vi "CRYPer.Rub& Buzz.vi"(4 "response":dbl[](array[numeric]), 5 "stimulus":dbl[](array[numeric]), 8 "cycle":dbl, 9 "frequency":dbl) -> (3 "out Y":dbl)   [LabVIEW 2013]
panel:
  in  "response 2":dbl[](array[numeric])
  in  "stimulus 2":dbl[](array[numeric])
  out "Array":dbl[](array[numeric])
  out "Version":i32
  out "Real matrix":dbl[][](array[numeric])
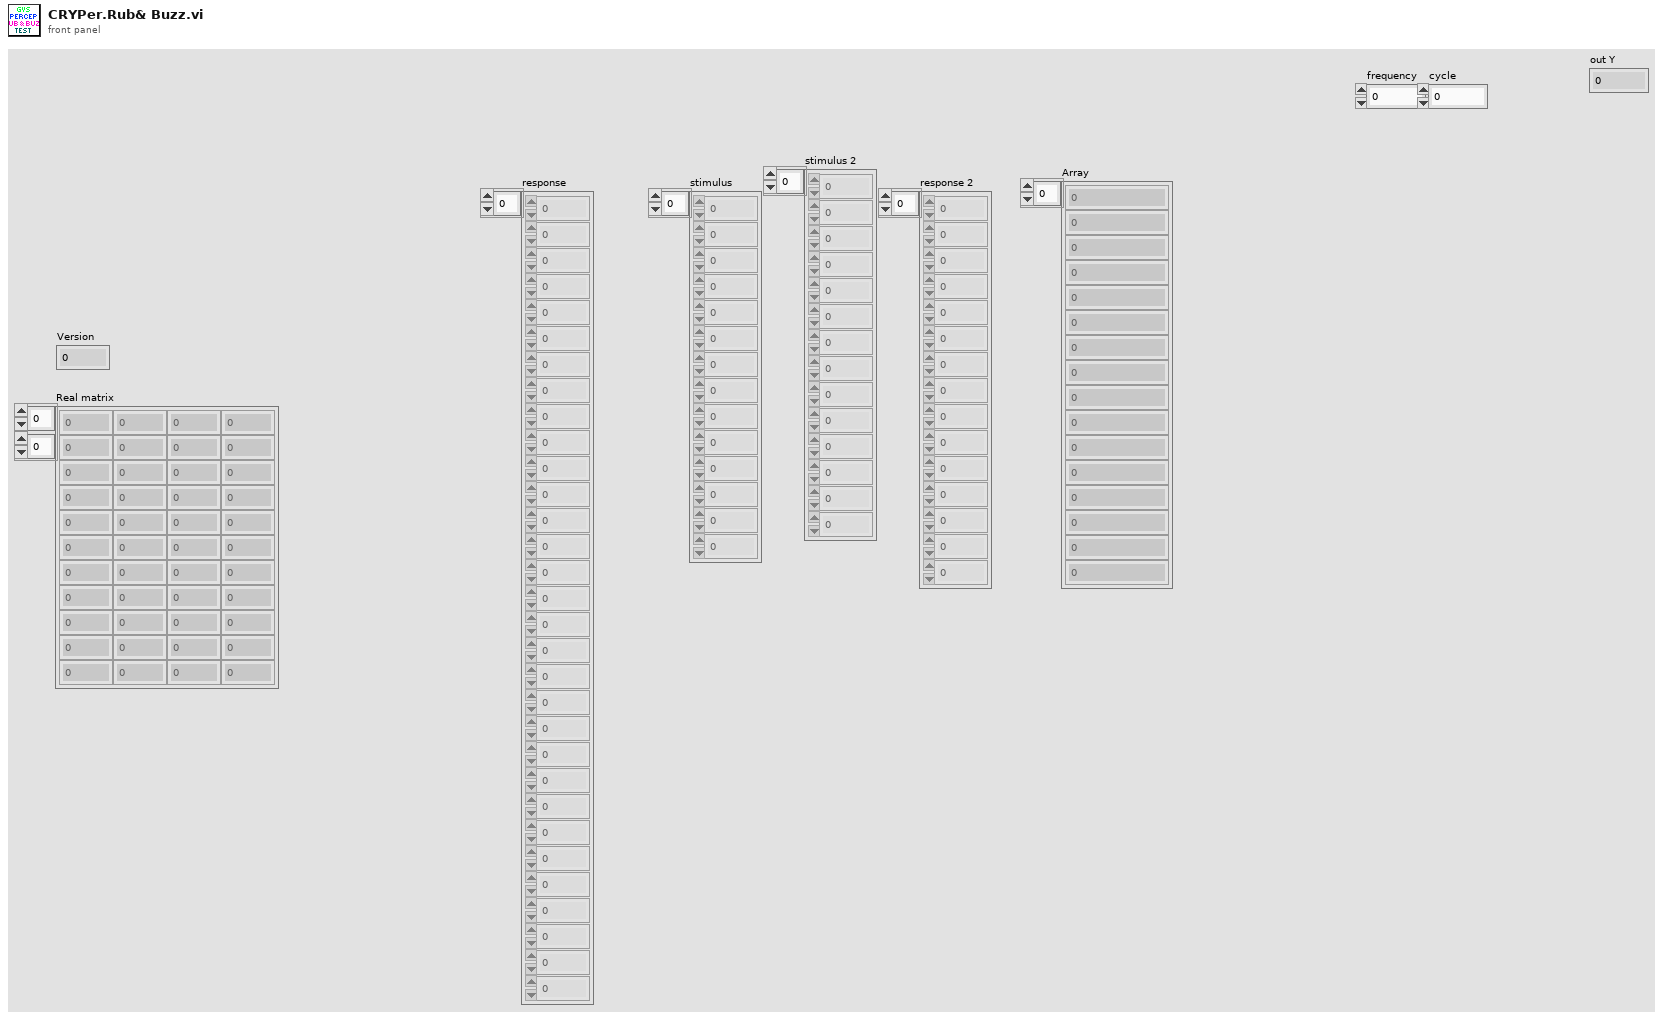
[diagram p1: front panel]
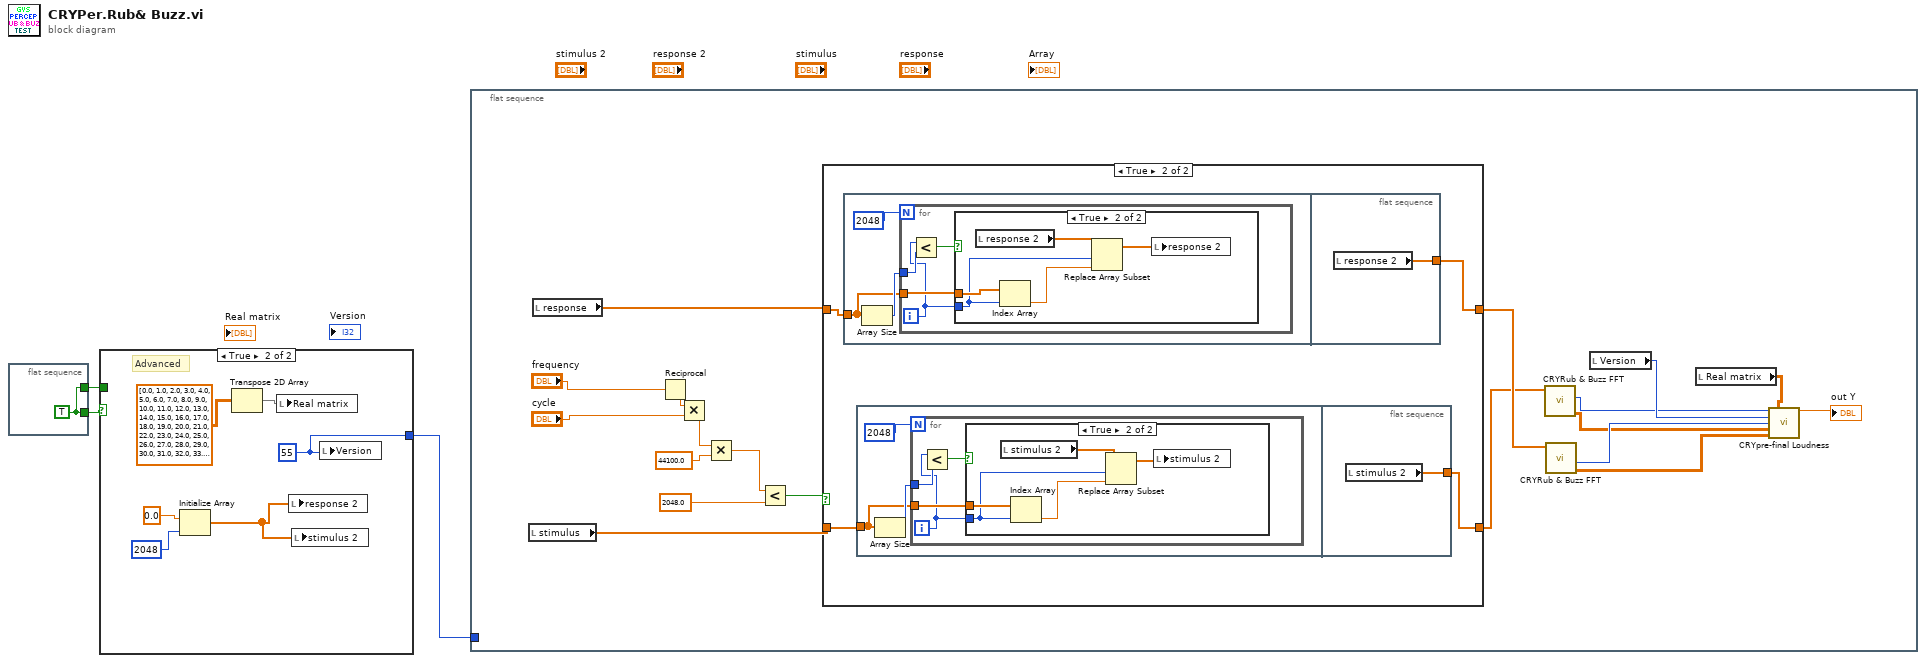
[diagram p0: block diagram]
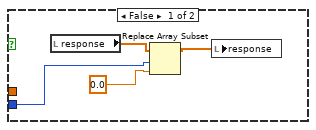
[diagram p3: hidden frame]
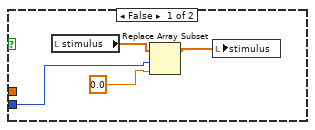
[diagram p4: hidden frame]
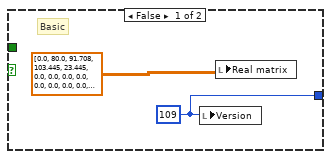
[diagram p5: hidden frame]
diagram:
  n1 = flat-sequence {
    tunnel: [w4] -> w3
    tunnel: [w4] -> w2
    frame #0 {
      w4 = TRUE
    }
  }
  n2 = case shown="True" w3 {
    tunnel: [w6 w12] -> w1
    tunnel: w2 -> [_ _]
    frame False {
      w6 = 109
      # "Basic"
      n3 = local write "Version"(w6) -> ()
      n4 = local write "Real matrix"(dbl[][] [[0.0, 80.0, 91.708, 103.445, 23.445, 0.0, 0.0, 0.0, 0.0, 0.0, 0.0, 0.0, 0.0, 0.0], [1.0, 103.445, 115.216, 127.023, 23.577, 0.0, 0.0, 0.0, 0.0, 0.0, 0.0, 0.0, 0.0, 0.0], [2.0, 127.023, 138.87, 150.762, 23.739, 0.0, 0.0, 0.0, 0.0, 0.0, 0.0, 0.0, 0.0, 0.0], [3.0, 150.762, 162.702, 174.694, 23.932, 0.0, 0.0, 0.0, 0.0, 0.0, 0.0, 0.0, 0.0, 0.0], [4.0, 174.694, 186.742, 198.849, 24.155, 0.0, 0.0, 0.0, 0.0, 0.0, 0.0, 0.0, 0.0, 0.0], [5.0, 198.849, 211.019, 223.257, 24.408, 0.0, 0.0, 0.0, 0.0, 0.0, 0.0, 0.0, 0.0, 0.0], [6.0, 223.257, 235.566, 247.95, 24.693, 0.0, 0.0, 0.0, 0.0, 0.0, 0.0, 0.0, 0.0, 0.0], [7.0, 247.95, 260.413, 272.959, 25.009, 0.0, 0.0, 0.0, 0.0, 0.0, 0.0, 0.0, 0.0, 0.0], [8.0, 272.959, 285.593, 298.317, 25.358, 0.0, 0.0, 0.0, 0.0, 0.0, 0.0, 0.0, 0.0, 0.0], [9.0, 298.317, 311.136, 324.055, 25.738, 0.0, 0.0, 0.0, 0.0, 0.0, 0.0, 0.0, 0.0, 0.0], [10.0, 324.055, 337.077, 350.207, 26.151, 0.0, 0.0, 0.0, 0.0, 0.0, 0.0, 0.0, 0.0, 0.0], [11.0, 350.207, 363.448, 376.805, 26.598, 0.0, 0.0, 0.0, 0.0, 0.0, 0.0, 0.0, 0.0, 0.0], [12.0, 376.805, 390.282, 403.884, 27.079, 0.0, 0.0, 0.0, 0.0, 0.0, 0.0, 0.0, 0.0, 0.0], [13.0, 403.884, 417.614, 431.478, 27.594, 0.0, 0.0, 0.0, 0.0, 0.0, 0.0, 0.0, 0.0, 0.0], [14.0, 431.478, 445.479, 459.622, 28.145, 0.0, 0.0, 0.0, 0.0, 0.0, 0.0, 0.0, 0.0, 0.0], [15.0, 459.622, 473.912, 488.353, 28.731, 0.0, 0.0, 0.0, 0.0, 0.0, 0.0, 0.0, 0.0, 0.0], [16.0, 488.353, 502.95, 517.707, 29.354, 0.0, 0.0, 0.0, 0.0, 0.0, 0.0, 0.0, 0.0, 0.0], [17.0, 517.707, 532.629, 547.721, 30.014, 0.0, 0.0, 0.0, 0.0, 0.0, 0.0, 0.0, 0.0, 0.0], [18.0, 547.721, 562.988, 578.434, 30.713, 0.0, 0.0, 0.0, 0.0, 0.0, 0.0, 0.0, 0.0, 0.0], [19.0, 578.434, 594.065, 609.885, 31.451, 0.0, 0.0, 0.0, 0.0, 0.0, 0.0, 0.0, 0.0, 0.0], [20.0, 609.885, 625.899, 642.114, 32.229, 0.0, 0.0, 0.0, 0.0, 0.0, 0.0, 0.0, 0.0, 0.0], [21.0, 642.114, 658.533, 675.161, 33.048, 0.0, 0.0, 0.0, 0.0, 0.0, 0.0, 0.0, 0.0, 0.0], [22.0, 675.161, 692.006, 709.071, 33.909, 0.0, 0.0, 0.0, 0.0, 0.0, 0.0, 0.0, 0.0, 0.0], [23.0, 709.071, 726.362, 743.884, 34.814, 0.0, 0.0, 0.0, 0.0, 0.0, 0.0, 0.0, 0.0, 0.0], [24.0, 743.884, 761.644, 779.647, 35.763, 0.0, 0.0, 0.0, 0.0, 0.0, 0.0, 0.0, 0.0, 0.0], [25.0, 779.647, 797.898, 816.404, 36.757, 0.0, 0.0, 0.0, 0.0, 0.0, 0.0, 0.0, 0.0, 0.0], [26.0, 816.404, 835.17, 854.203, 37.799, 0.0, 0.0, 0.0, 0.0, 0.0, 0.0, 0.0, 0.0, 0.0], [27.0, 816.404, 873.508, 893.091, 38.888, 0.0, 0.0, 0.0, 0.0, 0.0, 0.0, 0.0, 0.0, 0.0], [28.0, 893.091, 912.959, 933.119, 40.028, 0.0, 0.0, 0.0, 0.0, 0.0, 0.0, 0.0, 0.0, 0.0], [29.0, 933.119, 953.576, 974.336, 41.218, 0.0, 0.0, 0.0, 0.0, 0.0, 0.0, 0.0, 0.0, 0.0], [30.0, 974.336, 995.408, 1016.797, 42.461, 0.0, 0.0, 0.0, 0.0, 0.0, 0.0, 0.0, 0.0, 0.0], [31.0, 1016.797, 1038.511, 1060.555, 43.758, 0.0, 0.0, 0.0, 0.0, 0.0, 0.0, 0.0, 0.0, 0.0], [32.0, 1060.555, 1082.938, 1105.666, 45.111, 0.0, 0.0, 0.0, 0.0, 0.0, 0.0, 0.0, 0.0, 0.0], [33.0, 1105.666, 1128.746, 1152.187, 46.521, 0.0, 0.0, 0.0, 0.0, 0.0, 0.0, 0.0, 0.0, 0.0], [34.0, 1152.187, 1175.995, 1200.178, 47.991, 0.0, 0.0, 0.0, 0.0, 0.0, 0.0, 0.0, 0.0, 0.0], [35.0, 1200.178, 1224.744, 1249.7, 49.522, 0.0, 0.0, 0.0, 0.0, 0.0, 0.0, 0.0, 0.0, 0.0], [36.0, 1249.7, 1275.055, 1300.816, 51.116, 0.0, 0.0, 0.0, 0.0, 0.0, 0.0, 0.0, 0.0, 0.0], [37.0, 1300.816, 1326.992, 1353.592, 52.776, 0.0, 0.0, 0.0, 0.0, 0.0, 0.0, 0.0, 0.0, 0.0], [38.0, 1353.592, 1380.623, 1408.094, 54.502, 0.0, 0.0, 0.0, 0.0, 0.0, 0.0, 0.0, 0.0, 0.0], [39.0, 1408.094, 1436.014, 1464.392, 56.298, 0.0, 0.0, 0.0, 0.0, 0.0, 0.0, 0.0, 0.0, 0.0], [40.0, 1464.392, 1493.237, 1522.559, 58.167, 0.0, 0.0, 0.0, 0.0, 0.0, 0.0, 0.0, 0.0, 0.0], [41.0, 1522.559, 1552.366, 1582.668, 60.109, 0.0, 0.0, 0.0, 0.0, 0.0, 0.0, 0.0, 0.0, 0.0], [42.0, 1582.668, 1613.474, 1644.795, 62.128, 0.0, 0.0, 0.0, 0.0, 0.0, 0.0, 0.0, 0.0, 0.0], [43.0, 1644.795, 1676.641, 1709.021, 64.226, 0.0, 0.0, 0.0, 0.0, 0.0, 0.0, 0.0, 0.0, 0.0], [44.0, 1709.021, 1741.946, 1775.427, 66.406, 0.0, 0.0, 0.0, 0.0, 0.0, 0.0, 0.0, 0.0, 0.0], [45.0, 1775.427, 1809.474, 1844.098, 68.671, 0.0, 0.0, 0.0, 0.0, 0.0, 0.0, 0.0, 0.0, 0.0], [46.0, 1844.098, 1879.31, 1915.121, 71.023, 0.0, 0.0, 0.0, 0.0, 0.0, 0.0, 0.0, 0.0, 0.0], [47.0, 1915.121, 1951.543, 1988.587, 73.466, 0.0, 0.0, 0.0, 0.0, 0.0, 0.0, 0.0, 0.0, 0.0], [48.0, 1988.587, 2026.266, 2064.59, 76.003, 0.0, 0.0, 0.0, 0.0, 0.0, 0.0, 0.0, 0.0, 0.0], [49.0, 2064.59, 2103.573, 2143.217, 78.637, 0.0, 0.0, 0.0, 0.0, 0.0, 0.0, 0.0, 0.0, 0.0], [50.0, 2143.217, 2183.564, 2224.597, 81.371, 0.0, 0.0, 0.0, 0.0, 0.0, 0.0, 0.0, 0.0, 0.0], [51.0, 2224.597, 2266.34, 2308.806, 84.208, 0.0, 0.0, 0.0, 0.0, 0.0, 0.0, 0.0, 0.0, 0.0], [52.0, 2308.806, 2352.008, 2395.959, 87.154, 0.0, 0.0, 0.0, 0.0, 0.0, 0.0, 0.0, 0.0, 0.0], [53.0, 2395.959, 2440.675, 2486.169, 90.21, 0.0, 0.0, 0.0, 0.0, 0.0, 0.0, 0.0, 0.0, 0.0], [54.0, 2486.169, 2532.456, 2579.551, 93.382, 0.0, 0.0, 0.0, 0.0, 0.0, 0.0, 0.0, 0.0, 0.0], [55.0, 2579.551, 2627.468, 2676.223, 96.672, 0.0, 0.0, 0.0, 0.0, 0.0, 0.0, 0.0, 0.0, 0.0], [56.0, 2676.223, 2725.832, 2776.309, 100.086, 0.0, 0.0, 0.0, 0.0, 0.0, 0.0, 0.0, 0.0, 0.0], [57.0, 2776.309, 2827.672, 2879.937, 103.627, 0.0, 0.0, 0.0, 0.0, 0.0, 0.0, 0.0, 0.0, 0.0], [58.0, 2879.937, 2933.12, 2987.238, 107.302, 0.0, 0.0, 0.0, 0.0, 0.0, 0.0, 0.0, 0.0, 0.0], [59.0, 2987.238, 3042.309, 3098.35, 111.112, 0.0, 0.0, 0.0, 0.0, 0.0, 0.0, 0.0, 0.0, 0.0], [60.0, 3098.35, 3155.379, 3213.415, 115.065, 0.0, 0.0, 0.0, 0.0, 0.0, 0.0, 0.0, 0.0, 0.0], [61.0, 3213.415, 3272.475, 3332.579, 119.164, 0.0, 0.0, 0.0, 0.0, 0.0, 0.0, 0.0, 0.0, 0.0], [62.0, 3332.579, 3393.745, 3455.993, 123.415, 0.0, 0.0, 0.0, 0.0, 0.0, 0.0, 0.0, 0.0, 0.0], [63.0, 3455.993, 3519.344, 3583.817, 127.823, 0.0, 0.0, 0.0, 0.0, 0.0, 0.0, 0.0, 0.0, 0.0], [64.0, 3583.817, 3649.432, 3716.212, 132.395, 0.0, 0.0, 0.0, 0.0, 0.0, 0.0, 0.0, 0.0, 0.0], [65.0, 3716.212, 3784.176, 3853.348, 137.136, 0.0, 0.0, 0.0, 0.0, 0.0, 0.0, 0.0, 0.0, 0.0], [66.0, 3853.348, 3923.748, 3995.399, 142.051, 0.0, 0.0, 0.0, 0.0, 0.0, 0.0, 0.0, 0.0, 0.0], [67.0, 3995.399, 4068.324, 4142.547, 147.148, 0.0, 0.0, 0.0, 0.0, 0.0, 0.0, 0.0, 0.0, 0.0], [68.0, 4142.547, 4218.09, 4294.979, 152.432, 0.0, 0.0, 0.0, 0.0, 0.0, 0.0, 0.0, 0.0, 0.0], [69.0, 4294.979, 4373.237, 4452.89, 157.911, 0.0, 0.0, 0.0, 0.0, 0.0, 0.0, 0.0, 0.0, 0.0], [70.0, 4452.89, 4533.963, 4616.482, 163.592, 0.0, 0.0, 0.0, 0.0, 0.0, 0.0, 0.0, 0.0, 0.0], [71.0, 4616.482, 4700.473, 4785.962, 169.48, 0.0, 0.0, 0.0, 0.0, 0.0, 0.0, 0.0, 0.0, 0.0], [72.0, 4785.962, 4872.978, 4961.548, 175.585, 0.0, 0.0, 0.0, 0.0, 0.0, 0.0, 0.0, 0.0, 0.0], [73.0, 4961.548, 5051.7, 5143.463, 181.915, 0.0, 0.0, 0.0, 0.0, 0.0, 0.0, 0.0, 0.0, 0.0], [74.0, 5143.463, 5236.866, 5331.939, 188.476, 0.0, 0.0, 0.0, 0.0, 0.0, 0.0, 0.0, 0.0, 0.0], [75.0, 5331.939, 5428.712, 5527.217, 195.278, 0.0, 0.0, 0.0, 0.0, 0.0, 0.0, 0.0, 0.0, 0.0], [76.0, 5527.217, 5627.484, 5729.545, 202.329, 0.0, 0.0, 0.0, 0.0, 0.0, 0.0, 0.0, 0.0, 0.0], [77.0, 5729.545, 5833.434, 5939.183, 209.637, 0.0, 0.0, 0.0, 0.0, 0.0, 0.0, 0.0, 0.0, 0.0], [78.0, 5939.183, 6046.825, 6156.396, 217.214, 0.0, 0.0, 0.0, 0.0, 0.0, 0.0, 0.0, 0.0, 0.0], [79.0, 6156.396, 6267.931, 6381.463, 225.067, 0.0, 0.0, 0.0, 0.0, 0.0, 0.0, 0.0, 0.0, 0.0], [80.0, 6381.463, 6497.031, 6614.671, 233.208, 0.0, 0.0, 0.0, 0.0, 0.0, 0.0, 0.0, 0.0, 0.0], [81.0, 6614.671, 6734.42, 6856.316, 241.646, 0.0, 0.0, 0.0, 0.0, 0.0, 0.0, 0.0, 0.0, 0.0], [82.0, 6856.316, 6980.399, 7106.708, 250.392, 0.0, 0.0, 0.0, 0.0, 0.0, 0.0, 0.0, 0.0, 0.0], [83.0, 7106.708, 7235.284, 7366.166, 259.458, 0.0, 0.0, 0.0, 0.0, 0.0, 0.0, 0.0, 0.0, 0.0], [84.0, 7366.166, 7499.397, 7635.02, 268.854, 0.0, 0.0, 0.0, 0.0, 0.0, 0.0, 0.0, 0.0, 0.0], [85.0, 7635.02, 7773.077, 7913.614, 278.594, 0.0, 0.0, 0.0, 0.0, 0.0, 0.0, 0.0, 0.0, 0.0], [86.0, 7913.614, 8056.673, 8202.302, 288.688, 0.0, 0.0, 0.0, 0.0, 0.0, 0.0, 0.0, 0.0, 0.0], [87.0, 8202.302, 8350.547, 8501.454, 299.152, 0.0, 0.0, 0.0, 0.0, 0.0, 0.0, 0.0, 0.0, 0.0], [88.0, 8501.454, 8655.072, 8811.45, 309.996, 0.0, 0.0, 0.0, 0.0, 0.0, 0.0, 0.0, 0.0, 0.0], [89.0, 8811.45, 8970.639, 9132.688, 321.237, 0.0, 0.0, 0.0, 0.0, 0.0, 0.0, 0.0, 0.0, 0.0], [90.0, 9132.688, 9297.648, 9465.574, 332.887, 0.0, 0.0, 0.0, 0.0, 0.0, 0.0, 0.0, 0.0, 0.0], [91.0, 9465.574, 9636.52, 9810.536, 344.962, 0.0, 0.0, 0.0, 0.0, 0.0, 0.0, 0.0, 0.0, 0.0], [92.0, 9810.536, 9987.683, 10168.013, 357.477, 0.0, 0.0, 0.0, 0.0, 0.0, 0.0, 0.0, 0.0, 0.0], [93.0, 10168.013, 10351.586, 10538.46, 370.447, 0.0, 0.0, 0.0, 0.0, 0.0, 0.0, 0.0, 0.0, 0.0], [94.0, 10538.46, 10728.695, 10922.351, 383.891, 0.0, 0.0, 0.0, 0.0, 0.0, 0.0, 0.0, 0.0, 0.0], [95.0, 10922.351, 11119.49, 11320.175, 397.824, 0.0, 0.0, 0.0, 0.0, 0.0, 0.0, 0.0, 0.0, 0.0], [96.0, 11320.175, 11524.47, 11732.438, 412.264, 0.0, 0.0, 0.0, 0.0, 0.0, 0.0, 0.0, 0.0, 0.0], [97.0, 11732.438, 11944.149, 12159.67, 427.231, 0.0, 0.0, 0.0, 0.0, 0.0, 0.0, 0.0, 0.0, 0.0], [98.0, 12159.67, 12379.066, 12602.412, 442.742, 0.0, 0.0, 0.0, 0.0, 0.0, 0.0, 0.0, 0.0, 0.0], [99.0, 12602.412, 12829.775, 13061.229, 458.817, 0.0, 0.0, 0.0, 0.0, 0.0, 0.0, 0.0, 0.0, 0.0], [100.0, 13061.229, 13296.85, 13536.71, 475.48, 0.0, 0.0, 0.0, 0.0, 0.0, 0.0, 0.0, 0.0, 0.0], [101.0, 13536.71, 13780.887, 14029.458, 492.748, 0.0, 0.0, 0.0, 0.0, 0.0, 0.0, 0.0, 0.0, 0.0], [102.0, 14029.458, 14282.503, 14540.103, 510.645, 0.0, 0.0, 0.0, 0.0, 0.0, 0.0, 0.0, 0.0, 0.0], [103.0, 14540.103, 14802.338, 15069.295, 529.192, 0.0, 0.0, 0.0, 0.0, 0.0, 0.0, 0.0, 0.0, 0.0], [104.0, 15069.295, 15341.057, 15617.71, 548.415, 0.0, 0.0, 0.0, 0.0, 0.0, 0.0, 0.0, 0.0, 0.0], [105.0, 15617.71, 15899.345, 16186.049, 568.339, 0.0, 0.0, 0.0, 0.0, 0.0, 0.0, 0.0, 0.0, 0.0], [106.0, 16186.049, 16477.914, 16775.035, 588.986, 0.0, 0.0, 0.0, 0.0, 0.0, 0.0, 0.0, 0.0, 0.0], [107.0, 16775.035, 17077.504, 17385.42, 610.385, 0.0, 0.0, 0.0, 0.0, 0.0, 0.0, 0.0, 0.0, 0.0], [108.0, 17385.42, 17690.045, 18000.0, 614.58, 0.0, 0.0, 0.0, 0.0, 0.0, 0.0, 0.0, 0.0, 0.0]] ("Real matrix")) -> ()
    }
    frame True {
      w12 = 55
      # "Advanced"
      n5 = Initialize Array(0.0, 2048) -> (w9:dbl[])
      n6 = Transpose 2D Array(2D array=dbl[][] [[0.0, 1.0, 2.0, 3.0, 4.0, 5.0, 6.0, 7.0, 8.0, 9.0, 10.0, 11.0, 12.0, 13.0, 14.0, 15.0, 16.0, 17.0, 18.0, 19.0, 20.0, 21.0, 22.0, 23.0, 24.0, 25.0, 26.0, 27.0, 28.0, 29.0, 30.0, 31.0, 32.0, 33.0, 34.0, 35.0, 36.0, 37.0, 38.0, 39.0, 40.0, 41.0, 42.0, 43.0, 44.0, 45.0, 46.0, 47.0, 48.0, 49.0, 50.0, 51.0, 52.0, 53.0, 54.0, 0.0, 0.0, 0.0, 0.0, 0.0, 0.0, 0.0, 0.0, 0.0, 0.0, 0.0, 0.0, 0.0, 0.0, 0.0, 0.0, 0.0, 0.0, 0.0, 0.0, 0.0, 0.0, 0.0, 0.0, 0.0, 0.0, 0.0, 0.0, 0.0, 0.0, 0.0, 0.0, 0.0, 0.0, 0.0, 0.0, 0.0, 0.0, 0.0, 0.0, 0.0, 0.0, 0.0, 0.0, 0.0, 0.0, 0.0, 0.0, 0.0, 0.0, 0.0, 0.0, 0.0, 0.0], [80.00000000000004, 127.02285462585924, 174.69406062991834, 223.2569418786124, 272.9593735364518, 324.0550472730195, 376.80476615863523, 431.47777585810337, 488.3531389172424, 547.7211591568381, 609.8848634444312, 675.1615484072119, 743.884399980771, 816.4041940602248, 893.0910869341923, 974.3365046403833, 1060.5551408864565, 1152.1870737339648, 1249.700011849382, 1353.5916817875536, 1464.3923684927613, 1582.6676219846654, 1709.0211440446049, 1844.0978696365207, 1988.5872587907234, 2143.226815752958, 2308.8058533612657, 2486.1695218647915, 2676.2231227485, 2879.936729582437, 3098.350139481369, 3332.5781804480353, 3583.816401689871, 3853.347175953723, 4142.546245026183, 4452.889741809156, 4785.9617248128025, 5143.462263523483, 5527.216115916157, 5939.182042403041, 6381.462803758932, 6856.315894054644, 7366.165063381783, 7913.612689183225, 8501.45305933516, 9132.686634780404, 9810.535364512396, 10538.459131080843, 11320.173410560252, 12159.668237121652, 13061.228569006591, 14029.45615985561, 15069.293047027177, 16186.046776796207, 17385.417495187132, 0.0, 0.0, 0.0, 0.0, 0.0, 0.0, 0.0, 0.0, 0.0, 0.0, 0.0, 0.0, 0.0, 0.0, 0.0, 0.0, 0.0, 0.0, 0.0, 0.0, 0.0, 0.0, 0.0, 0.0, 0.0, 0.0, 0.0, 0.0, 0.0, 0.0, 0.0, 0.0, 0.0, 0.0, 0.0, 0.0, 0.0, 0.0, 0.0, 0.0, 0.0, 0.0, 0.0, 0.0, 0.0, 0.0, 0.0, 0.0, 0.0, 0.0, 0.0, 0.0, 0.0, 0.0], [103.44500000000002, 150.7618443751613, 198.8482089273687, 247.94953657964493, 298.3164508402441, 350.20603503777454, 403.8831445286032, 459.62175857432595, 517.7063787895687, 578.433481298095, 642.1130300093238, 709.0700587393488, 779.646330251927, 854.2020806875403, 933.1178582844567, 1016.7964657770141, 1105.6650163855336, 1200.1771138920699, 1300.8151679295622, 1408.092856302109, 1522.557746904569, 1644.7940926243168, 1775.4258134909153, 1915.1196812952376, 2064.5887229329837, 2224.5958598439975, 2395.9578021238235, 2579.549217183894, 2776.30719423804, 2987.2360274030216, 3213.4123418270237, 3455.9905890109603, 3716.2089393718493, 3995.3956021251624, 4294.975604744136, 4616.4780665998605, 4961.544003908298, 5331.934705822349, 5729.540724422322, 6156.391524491527, 6614.665842331607, 7106.702806491036, 7635.01387716947, 8202.29566523903, 8811.443696313632, 9465.567190121013, 10168.004930614432, 10922.342307828547, 11732.429618464565, 12602.40171861481, 13536.69912893825, 14540.090700012326, 15617.69795354979, 16775.021223723146, 17690.045, 0.0, 0.0, 0.0, 0.0, 0.0, 0.0, 0.0, 0.0, 0.0, 0.0, 0.0, 0.0, 0.0, 0.0, 0.0, 0.0, 0.0, 0.0, 0.0, 0.0, 0.0, 0.0, 0.0, 0.0, 0.0, 0.0, 0.0, 0.0, 0.0, 0.0, 0.0, 0.0, 0.0, 0.0, 0.0, 0.0, 0.0, 0.0, 0.0, 0.0, 0.0, 0.0, 0.0, 0.0, 0.0, 0.0, 0.0, 0.0, 0.0, 0.0, 0.0, 0.0, 0.0, 0.0], [127.02299999999995, 174.69420836830608, 223.25709273533505, 272.9595282815137, 324.0552066962722, 376.80493107380823, 431.4779471069587, 488.35331737387, 547.7213457321184, 609.8850590906835, 675.1617541230561, 743.8846168162241, 816.4044231220599, 893.0913293915901, 974.3367617308965, 1060.5554139223295, 1152.18736410883, 1249.7003210453747, 1353.5920113828745, 1464.3927201697347, 1582.6679975383238, 1709.0215453918531, 1844.0982988259204, 1988.5877180129467, 2143.2273073519727, 2308.8063798462963, 2486.170085923128, 2676.2237272592147, 2879.9373776310817, 3098.3508343757176, 3332.578925734977, 3583.8172011735082, 3853.348033714785, 4142.547165442865, 4452.890729579458, 4785.96278497851, 5143.463401495909, 5527.217337503748, 5939.183353841042, 6381.464211741191, 6856.317405767803, 7366.166686541948, 7913.61443207534, 8501.454930855318, 9132.688644481233, 9810.53752265184, 10538.461448674487, 11320.17589943759, 12159.670909986446, 13061.231439501691, 14029.459242632638, 15069.296357821262, 16186.050332506353, 17385.421313962415, 18000.0, 0.0, 0.0, 0.0, 0.0, 0.0, 0.0, 0.0, 0.0, 0.0, 0.0, 0.0, 0.0, 0.0, 0.0, 0.0, 0.0, 0.0, 0.0, 0.0, 0.0, 0.0, 0.0, 0.0, 0.0, 0.0, 0.0, 0.0, 0.0, 0.0, 0.0, 0.0, 0.0, 0.0, 0.0, 0.0, 0.0, 0.0, 0.0, 0.0, 0.0, 0.0, 0.0, 0.0, 0.0, 0.0, 0.0, 0.0, 0.0, 0.0, 0.0, 0.0, 0.0, 0.0, 0.0]] ("Array 2")) -> (transposed array=w10:dbl[][])
      n7 = local write "Real matrix"(w10) -> ()
      n8 = local write "response 2"(w9) -> ()
      n9 = local write "stimulus 2"(w9) -> ()
      n10 = local write "Version"(w12) -> ()
    }
  }
  n11 = flat-sequence {
    tunnel: w1 -> [_]
    frame #0 {
      n12 = local read "stimulus"() -> (w13:dbl[])
      n13 = local read "response"() -> (w14:dbl[])
      n14 = Reciprocal(x="frequency") -> (1/x=w29:dbl)
      n15 = Multiply(x=w29, y="cycle") -> (x*y=w28:dbl)
      n16 = Multiply(x=w28, y=44100.0 ("scaled")) -> (x*y=w18:dbl)
      n17 = Less?(x=w18, y=2048.0) -> (x < y?=w21:bool)
      n18 = case shown="True" w21 {
        tunnel: w13 -> [w32 w37]
        tunnel: w14 -> [w33 w36]
        tunnel: [w33 w35] -> w20
        tunnel: [w32 w34] -> w19
        frame False {
        }
        frame True {
          n19 = flat-sequence {
            tunnel: w36 -> [w38]
            tunnel: [w54] -> w35
            frame #0 {
              n20 = Array Size(array=w38) -> (size(s)=w39:i32)
              n21 = for {
                N: 2048 -> [_]
                tunnel: w38 -> [w44]
                tunnel: w39 -> [w43]
                i -> [w41]
                n22 = Less?(x=w41, y=w43) -> (x < y?=w42:bool)
                n23 = case shown="True" w42 {
                  tunnel: w44 -> [_ w53]
                  tunnel: w41 -> [w48 w49]
                  frame False {
                    n24 = local read "response"() -> (w47:dbl[])
                    n25 = Replace Array Subset(array=w47, new element=0.0, index=w48) -> (w46:dbl[])
                    n26 = local write "response"(w46) -> ()
                  }
                  frame True {
                    n27 = local read "response 2"() -> (w52:dbl[])
                    n28 = Index Array(array=w53, index=w49) -> (element=w51:dbl)
                    n29 = Replace Array Subset(array=w52, new element=w51, index=w49) -> (w50:dbl[])
                    n30 = local write "response 2"(w50) -> ()
                  }
                }
              }
            }
            frame #1 {
              n31 = local read "response 2"() -> (w54:dbl[])
            }
          }
          n32 = flat-sequence {
            tunnel: w37 -> [w55]
            tunnel: [w71] -> w34
            frame #0 {
              n33 = Array Size(array=w55) -> (size(s)=w56:i32)
              n34 = for {
                N: 2048 -> [_]
                tunnel: w55 -> [w61]
                tunnel: w56 -> [w60]
                i -> [w58]
                n35 = Less?(x=w58, y=w60) -> (x < y?=w59:bool)
                n36 = case shown="True" w59 {
                  tunnel: w61 -> [_ w70]
                  tunnel: w58 -> [w65 w66]
                  frame False {
                    n37 = local read "stimulus"() -> (w64:dbl[])
                    n38 = Replace Array Subset(array=w64, new element=0.0, index=w65) -> (w63:dbl[])
                    n39 = local write "stimulus"(w63) -> ()
                  }
                  frame True {
                    n40 = local read "stimulus 2"() -> (w69:dbl[])
                    n41 = Index Array(array=w70, index=w66) -> (element=w68:dbl)
                    n42 = Replace Array Subset(array=w69, new element=w68, index=w66) -> (w67:dbl[])
                    n43 = local write "stimulus 2"(w67) -> ()
                  }
                }
              }
            }
            frame #1 {
              n44 = local read "stimulus 2"() -> (w71:dbl[])
            }
          }
        }
      }
      n45 = call "CRYRub & Buzz FFT.vi"("wave data"=w19) -> ("Fe[n,kf]"=w24:dbl[][], "Frame number"=w23:i32)  [unwired: 7 in, 2 out]
      n46 = call "CRYRub & Buzz FFT.vi"("wave data"=w20) -> ("Fe[n,kf]"=w26:dbl[][], "size"=w25:i32)  [unwired: 7 in, 2 out]
      n47 = local read "Version"() -> (w27:i32)
      n48 = local read "Real matrix"() -> (w30:dbl[][])
      n49 = call "CRYpre-final Loudness.vi"("Frame number"=w23, "Real matrix"=w30, "Version"=w27, "size"=w25, "Fe(stim)[n,kf]"=w24, "Fe(res)[n,kf]"=w26) -> ("total Loudness"=→"out Y":dbl)  [unwired: 9 in]
    }
  }
